vi "Sub-vi.vi"(1 "Compounded":string(combo), 2 "Year":dbl min=0.0 max=100.0, 3 "Interest rate":dbl format="%.2f%", 4 "Investment":dbl format="$%#_g") -> (0 "Final Amount":dbl format="$%#_g")   [LabVIEW 2020]
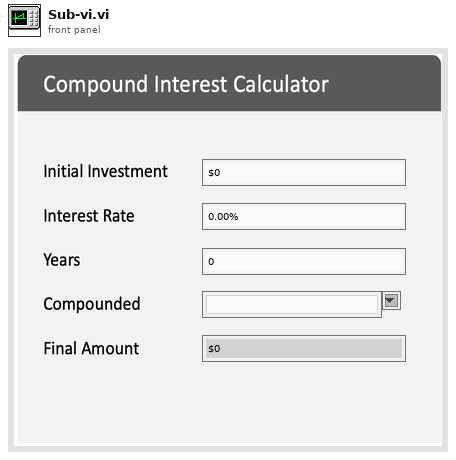
[diagram p1: front panel]
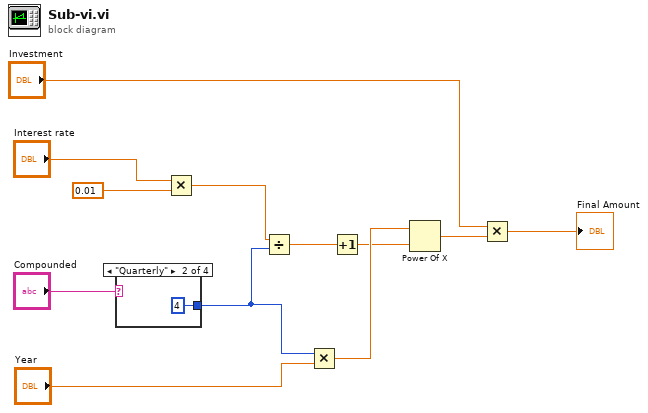
[diagram p0: block diagram]
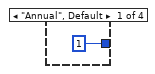
[diagram p2: hidden frame]
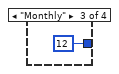
[diagram p3: hidden frame]
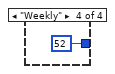
[diagram p4: hidden frame]
diagram:
  n1 = case shown="\"Quarterly\"" "Compounded" {
    tunnel: [1 4 12 52] -> w9
    frame "Annual", Default {
    }
    frame "Quarterly" {
    }
    frame "Monthly" {
    }
    frame "Weekly" {
    }
  }
  n2 = Multiply(x="Interest rate", y=0.01) -> (x*y=w3:dbl)
  n3 = Divide(x=w3, y=w9) -> (x/y=w11:dbl)
  n4 = Multiply(x=w9, y="Year") -> (x*y=w2:dbl)
  n5 = Increment(x=w11) -> (x+1=w1:dbl)
  n6 = Power Of X(1:w1, 2:w2) -> (0:w8:dbl)
  n7 = Multiply(x="Investment", y=w8) -> (x*y=→"Final Amount":dbl)
